vi "Insight_Create_Valid_Vector.vi"(8 "error in (no error)":errorcluster, 10 "Invalid Data Indices":i32[](array[numeric]), 11 "total data length":i32) -> (0 "error out":errorcluster, 2 "Valid Vector":i32[](array[numeric]))   [LabVIEW 2015]
doc: "Insight Photonic Solutions - v1.0\n\nThis VI creates a vector of indices (the \"Valid Vector\") for the Valid measurements in a sweep of the Insight laser, based on the Total Data Length and an array of Invalid Data Indices.\n\nUse this VI in combination with \"Insight_Reduce_Data_with_Valid-Vector\"."
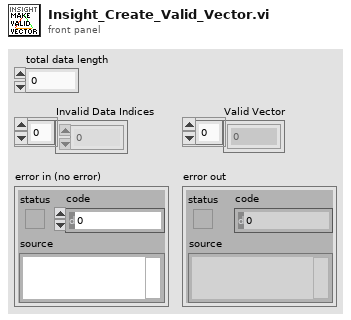
[diagram p1: front panel]
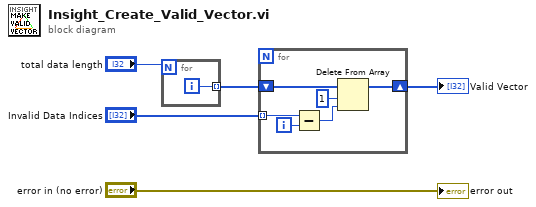
[diagram p0: block diagram]
diagram:
  n1 = for {
    N: "total data length" -> [_]
    tunnel: [w6] -> w5 mode=indexing
    i -> [w6]
  }
  n2 = for {
    tunnel: "Invalid Data Indices" -> [w9] mode=indexing
    shift-right: [w11] -> w3
    shift-left: w5 -> [w12]
    i -> [w8]
    n3 = Subtract(x=w9, y=w8) -> (x-y=w7:i32)
    n4 = Delete From Array(array=w12, length=1, index=w7) -> (array with subset deleted=w11:i32[])  [unwired: 1 out]
  }
  "Valid Vector" <- w3
  "error out" <- "error in (no error)"
